vi "子界面-图像预处理.vi"(11 "原图":T1(plugin-control)) -> (3 "处理后":T1(plugin-control))   [LabVIEW 2018]
uses:
  <vilib>/vision/NI_Vision_Development_Module.lvlib
panel:
  in  "模式选择":u16(ring) items=["AutoM", "Close", "Dilate", "Erode", "Gradient", "Gradient in", "Gradient out", "HitMiss", "Open", "PClose", "POpen", "Thick", "Thin"]
  in  "返回":bool
  in  "确认":bool
  in  "结构元素":dbl[][](array[numeric])
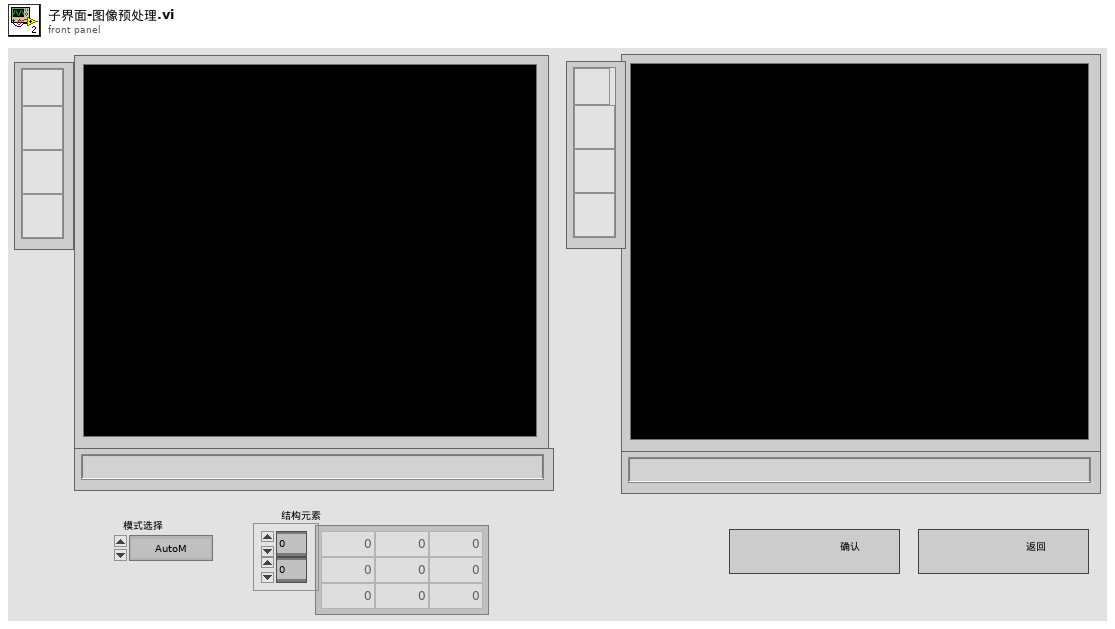
[diagram p1: front panel]
types:
  T1 = typedef "IMAQ Image.ctl" = refnum<image>
  T2 = typedef "Image Type" = u32
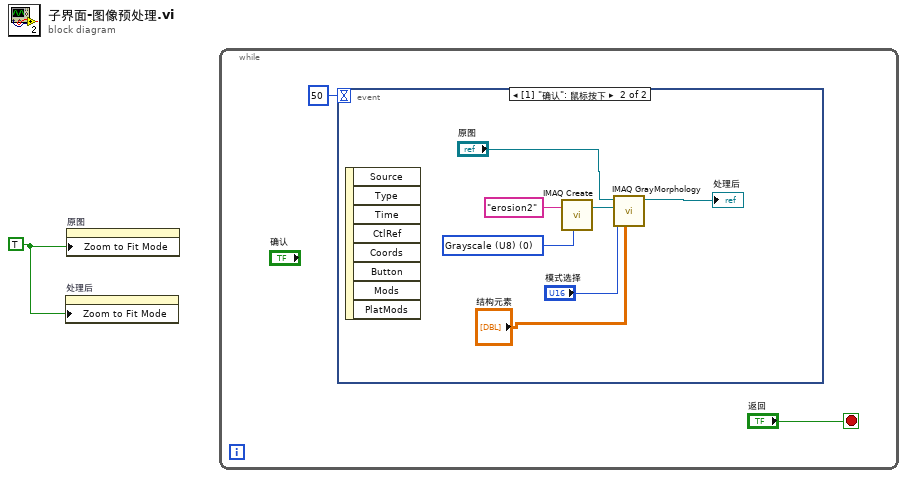
[diagram p0: block diagram]
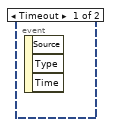
[diagram p2: hidden frame]
diagram:
  w1 = TRUE ("Zoom to Fit Mode")
  n1 = property on="处理后" class="ImageControl"("Zoom to Fit Mode"=w1) -> ()  [unwired: 2 in, 2 out]
  n2 = property on="原图" class="ImageControl"("Zoom to Fit Mode"=w1) -> ()  [unwired: 2 in, 2 out]
  n3 = while {
    stop <- "返回" stop-if-true
    n4 = event shown="[1] \"确认\": 鼠标按下" {
      selector: _ -> [_ _]
      dyn-events: _ -> [_ _]
      timeout: 50 -> [_ _]
      event Timeout {
        n5 = event-data() -> ()  [unwired: 1 in, 3 out]
      }
      event "确认": Mouse Down {
        w7 = T2 0 items=["Grayscale (U8)", "Grayscale (I16)", "Grayscale (SGL)", "Complex (CSG)", "RGB (U32)", "HSL (U32)", "RGB (U64)", "Grayscale (U16)"] ("Image Type")
        n6 = event-data() -> ()  [unwired: 1 in, 8 out]
        n7 = call "IMAQ Create"("Image Name"="erosion2", "Image Type"=w7) -> ("New Image"=w9:T1)  [unwired: 3 in, 1 out]
        n8 = call "IMAQ GrayMorphology"("Structuring Element"="结构元素", "Operation"="模式选择", "Image Dst"=w9, "Image Src"="原图") -> ("Image Dst Out"=→"处理后":T1)  [unwired: 6 in, 1 out]
      }
    }
  }
